vi "Build Ring.vi"(8 "error in (no error)":errorcluster, 10 "variant":variant, 11 "Ring":refnum<vi>) -> (0 "error out":errorcluster, 2 "duplicate variant":variant)   [LabVIEW 2023, in "J1939 Workspace Shared.lvlib"]
uses:
  J1939 Workspace Shared.lvlib
  Addon/Addon Shared/Types/Address Lookup Table Data.ctl
  Addon/Addon Shared/J1939 Addon Shared.lvlib
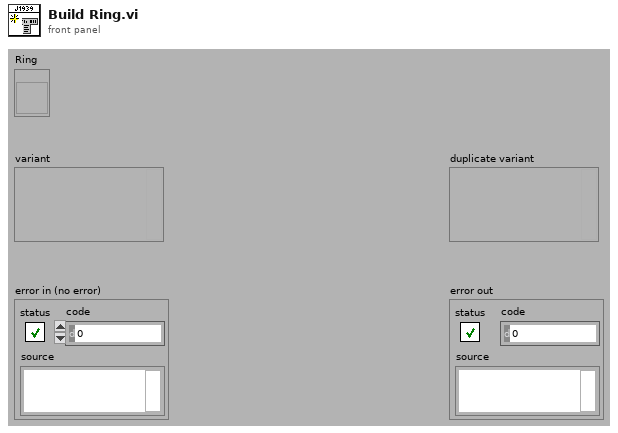
[diagram p1: front panel]
types:
  T1 = typedef "J1939 Addon Shared.lvlib/Address Lookup Table Data.ctl" = cluster{"Name":u8[], "Address":u8}
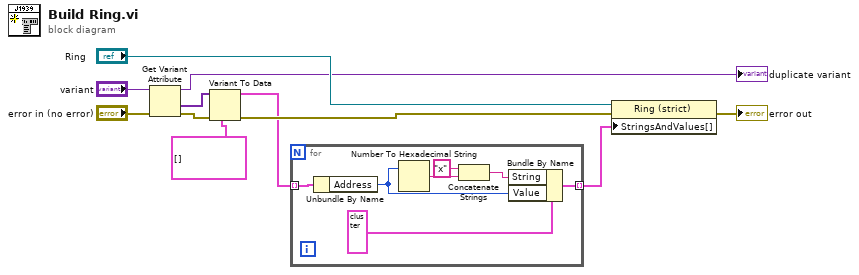
[diagram p0: block diagram]
diagram:
  n1 = Get Variant Attribute(Variant="variant", error in="error in (no error)") -> (duplicate Variant=→"duplicate variant":variant, values=w10:variant[], error out=w11:errorcluster)  [unwired: 2 in, 1 out]
  n2 = Variant To Data(error in=w11, type=T1[] [], Variant=w10) -> (data=w4:T1[], error out=w5:errorcluster)
  n3 = for {
    tunnel: w4 -> [w18] mode=indexing
    tunnel: [w16] -> w3 mode=indexing
    n4 = Unbundle By Name(w18) -> ("Address"=w15:u8)
    n5 = Number To Hexadecimal String(2:w15) -> (0:w14:string)  [unwired: 1 in]
    n6 = Concatenate Strings("x" ("string"), w14) -> (w13:string)
    n7 = Bundle By Name(cluster=cluster{"String":string, "Value":ext} {"String"="", "Value"=0.0}, "String"=w13, "Value"=w15) -> (w16:cluster{"String":string, "Value":ext})
  }
  n8 = property on="Property Node" class="Ring (strict)"(reference="Ring", error in=w5, "StringsAndValues[]"=w3) -> (error out=→"error out":errorcluster)  [unwired: 1 out]
